vi "connect to arduino.vi"() -> ()   [LabVIEW 2020]
uses:
  <vilib>/Instr/_visa.llb/VISA Configure Serial Port (Instr).vi
panel:
  in  "mesurement period (ms)":dbl(slide) scale=0.0..2000.0
  out "console":string
  in  "Connection":bool
  out "Connection LED":bool
  in  "baud rate (9600)":u32=9600
  out "Waveform Chart":dbl(graph)
  in  "Voltage mesure":bool
  in  "Single voltage":bool
  in  "LED blink":bool
  in  "LED on/off":bool
  out "Voltage":dbl
  in  "VISA 1":refnum<visa-resource-name>
  in  "exit":bool
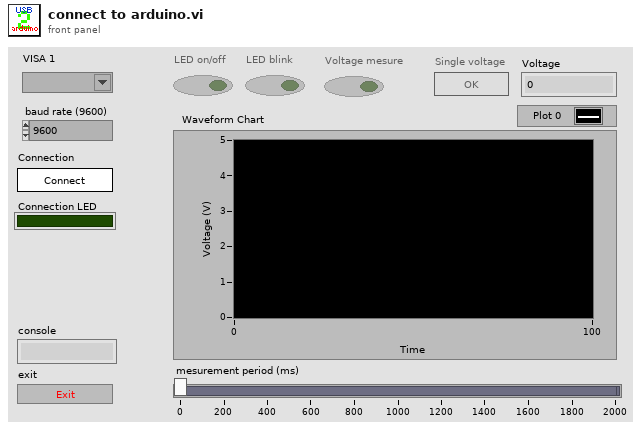
[diagram p1: front panel]
types:
  T1 = enum8{"Enabled", "Disabled", "Disabled and Grayed Out"}
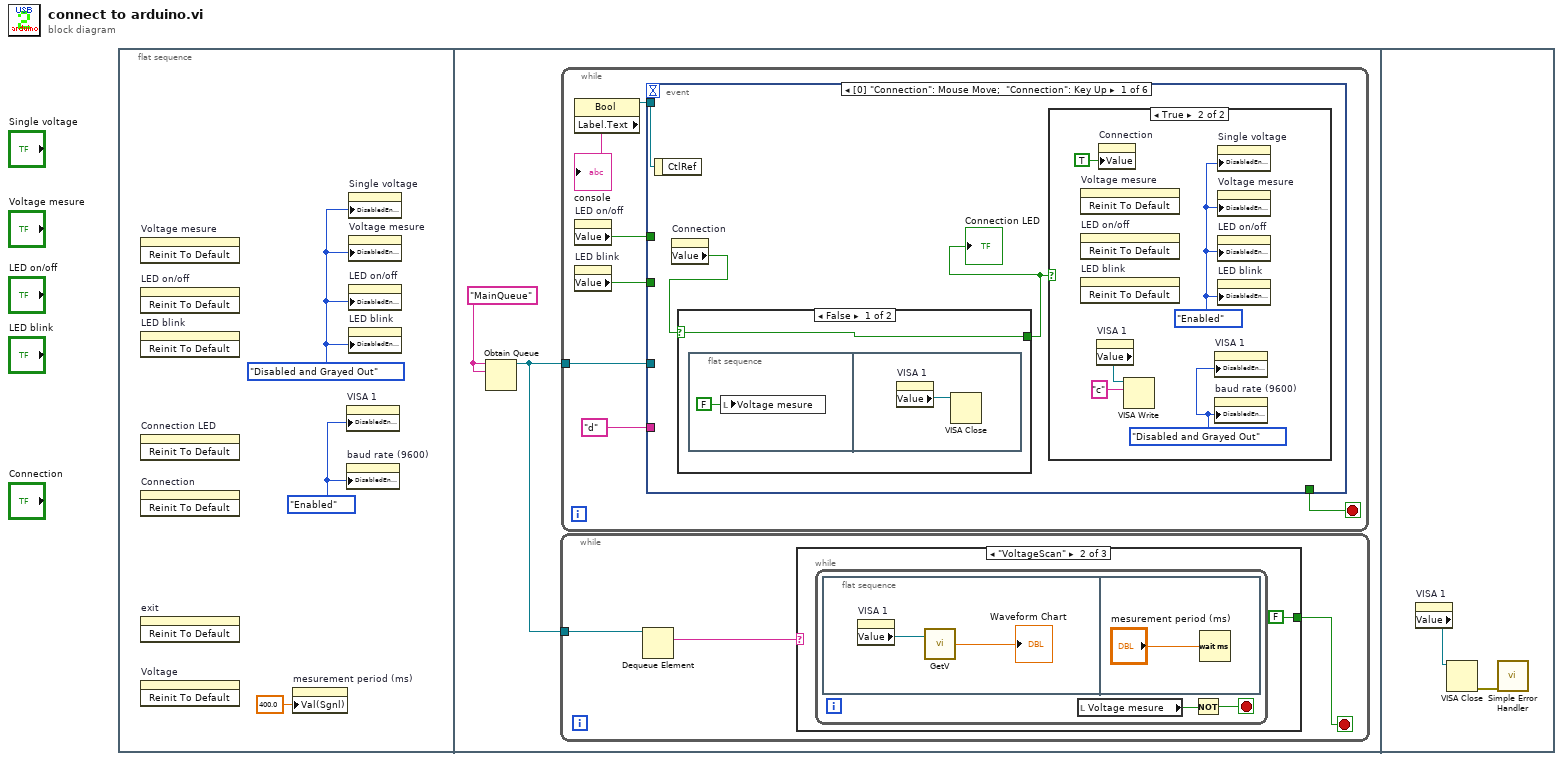
[diagram p0: block diagram]
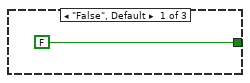
[diagram p2: hidden frame]
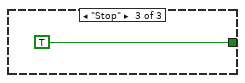
[diagram p3: hidden frame]
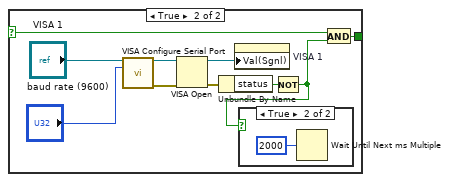
[diagram p4: hidden frame]
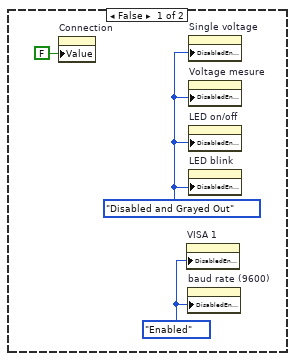
[diagram p6: hidden frame]
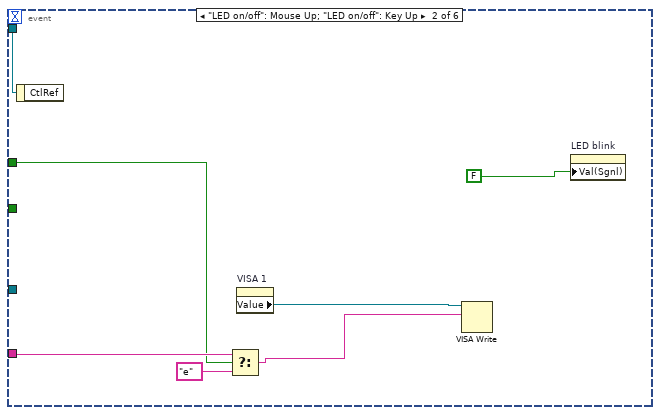
[diagram p7: hidden frame]
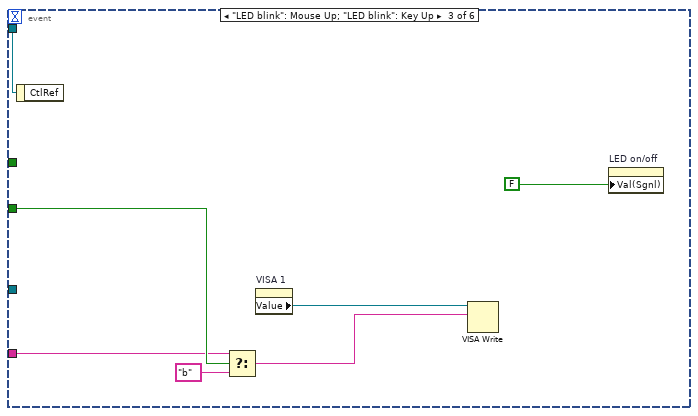
[diagram p8: hidden frame]
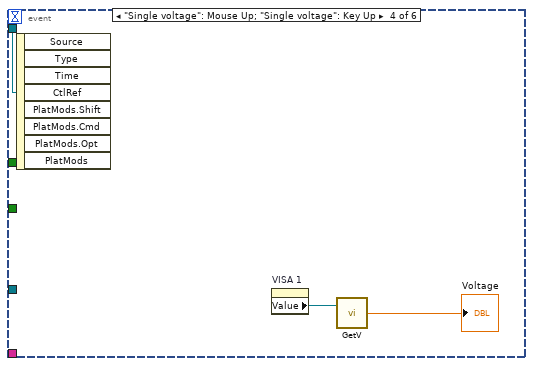
[diagram p9: hidden frame]
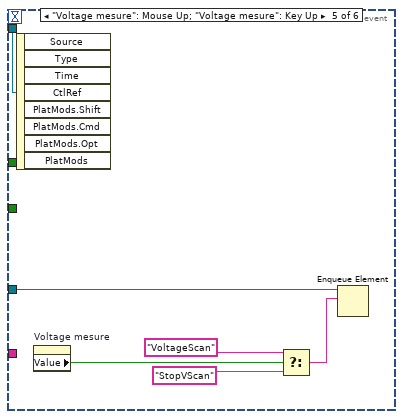
[diagram p10: hidden frame]
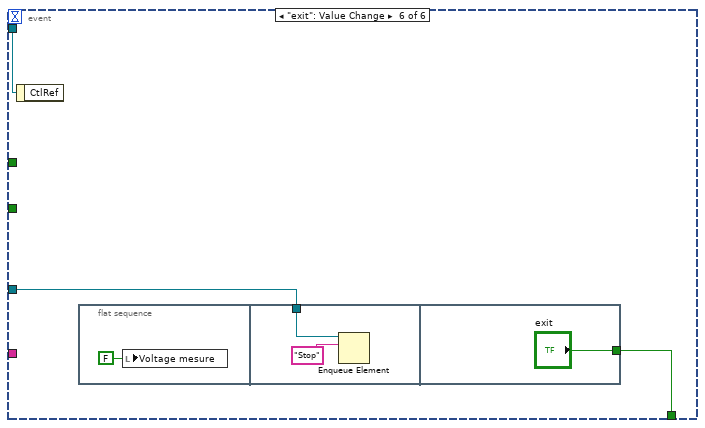
[diagram p11: hidden frame]
diagram:
  n1 = flat-sequence {
    frame #0 {
      w3 = T1."Enabled" ("Disabled")
      w2 = T1."Disabled and Grayed Out" ("Disabled")
      n2 = invoke on="Voltage mesure" class="Bool (strict)" method="Reinit To Default"() -> ()  [unwired: 3 in, 3 out]
      n3 = invoke on="LED on/off" class="Bool (strict)" method="Reinit To Default"() -> ()  [unwired: 3 in, 3 out]
      n4 = invoke on="LED blink" class="Bool (strict)" method="Reinit To Default"() -> ()  [unwired: 3 in, 3 out]
      n5 = invoke on="Connection LED" class="Bool (strict)" method="Reinit To Default"() -> ()  [unwired: 3 in, 3 out]
      n6 = invoke on="Connection" class="Bool (strict)" method="Reinit To Default"() -> ()  [unwired: 3 in, 3 out]
      n7 = invoke on="exit" class="Bool" method="Reinit To Default"() -> ()  [unwired: 3 in, 3 out]
      n8 = invoke on="Voltage" class="DigNum (strict)" method="Reinit To Default"() -> ()  [unwired: 3 in, 3 out]
      n9 = property on="mesurement period (ms)" class="Slide (strict)"("Val(Sgnl)"=400.0 ("Value (Signaling)")) -> ()  [unwired: 2 in, 2 out]
      n10 = property on="VISA 1" class="VISAName"("DisabledEnum"=w3) -> ()  [unwired: 2 in, 2 out]
      n11 = property on="baud rate (9600)" class="DigNum (strict)"("DisabledEnum"=w3) -> ()  [unwired: 2 in, 2 out]
      n12 = property on="Single voltage" class="Bool (strict)"("DisabledEnum"=w2) -> ()  [unwired: 2 in, 2 out]
      n13 = property on="Voltage mesure" class="Bool (strict)"("DisabledEnum"=w2) -> ()  [unwired: 2 in, 2 out]
      n14 = property on="LED on/off" class="Bool (strict)"("DisabledEnum"=w2) -> ()  [unwired: 2 in, 2 out]
      n15 = property on="LED blink" class="Bool (strict)"("DisabledEnum"=w2) -> ()  [unwired: 2 in, 2 out]
    }
    frame #1 {
      w5 = "MainQueue" ("name (unnamed)")
      n16 = Obtain Queue(name (unnamed)=w5, element data type=w5) -> (queue out=w4:refnum<queue>)  [unwired: 3 in, 2 out]
      n17 = while {
        tunnel: w4 -> [w6]
        stop <- w7 stop-if-true
        n18 = Dequeue Element(queue=w6) -> (element=w8:string)  [unwired: 2 in, 3 out]
        n19 = case shown="\"VoltageScan\"" w8 {
          tunnel: [FALSE FALSE TRUE] -> w7
          frame "False", Default {
          }
          frame "VoltageScan" {
            n20 = while {
              stop <- w12 stop-if-true
              n21 = flat-sequence {
                frame #0 {
                  n22 = property on="VISA 1" class="VISAName"() -> ("Value"=w13:refnum<visa-resource-name>)  [unwired: 2 in, 2 out]
                  n23 = call "GetV.vi"("VISA resource name"=w13) -> ("output 1"=→"Waveform Chart":dbl)  [unwired: 2 in, 1 out]
                }
                frame #1 {
                  n24 = Wait (ms)(milliseconds to wait="mesurement period (ms)") -> ()  [unwired: 1 out]
                }
              }
              n25 = local read "Voltage mesure"() -> (w11:bool)
              n26 = Not(x=w11) -> (.not. x?=w12:bool)
            }
          }
          frame "Stop" {
          }
        }
      }
      n27 = while {
        tunnel: w4 -> [w18]
        stop <- w17 stop-if-true
        n28 = property on="LED on/off" class="Bool (strict)"() -> ("Value"=w22:bool)  [unwired: 2 in, 2 out]
        n29 = property on="LED blink" class="Bool (strict)"() -> ("Value"=w21:bool)  [unwired: 2 in, 2 out]
        n30 = event shown="[0] \"Connection\": Mouse Move;  \"Connection\": Key Up" {
          selector: _ -> [_ _ _ _ _ _]
          dyn-events: _ -> [_ _ _ _ _ _]
          timeout: _ -> [_ _ _ _ _ _]
          tunnel: w22 -> [_ w52 _ _ _ _]
          tunnel: w21 -> [_ _ w61 _ _ _]
          tunnel: "d" -> [_ w54 w60 _ _ _]
          tunnel: [w26 w50 w57 w64 w70 w74] -> w19
          tunnel: [_ _ _ _ _ w73] -> w17
          tunnel: w18 -> [_ _ _ _ w71 w72]
          event "Connection": Mouse Move; "Connection": Key Up {
            n31 = event-data() -> ("CtlRef"=w26:refnum<vi>)  [unwired: 1 in]
            n32 = property on="Connection" class="Bool (strict)"() -> ("Value"=w25:bool)  [unwired: 2 in, 2 out]
            n33 = case shown="False" w25 {
              selector: w25 -> [w27 w33]
              tunnel: [w27 w34] -> w24
              frame False {
                n34 = flat-sequence {
                  frame #0 {
                    n35 = local write "Voltage mesure"(FALSE ("Voltage mesure")) -> ()
                  }
                  frame #1 {
                    n36 = property on="VISA 1" class="VISAName"() -> ("Value"=w29:refnum<visa-resource-name>)  [unwired: 2 in, 2 out]
                    n37 = VISA Close(VISA resource name=w29) -> ()  [unwired: 1 in, 1 out]
                  }
                }
              }
              frame True {
                n38 = call-poly "VISA Configure Serial Port"("VISA resource name"="VISA 1", "baud rate (9600)"="baud rate (9600)") -> ("VISA resource name out"=w36:refnum<visa-resource-name>, "error out"=w37:errorcluster)  [unwired: 12 in]
                n39 = VISA Open(error in (no error)=w37, VISA resource name=w36) -> (VISA resource name=w35:refnum<visa-resource-name>, error out=w31:errorcluster)  [unwired: 3 in]
                n40 = Unbundle By Name(w31) -> ("status"=w32:bool)
                n41 = property on="VISA 1" class="VISAName"("Val(Sgnl)"=w35) -> ()  [unwired: 2 in, 2 out]
                n42 = Not(x=w32) -> (.not. x?=w30:bool)
                n43 = case shown="True" w30 {
                  frame False {
                  }
                  frame True {
                    n44 = Wait Until Next ms Multiple(millisecond multiple=u32 2000) -> ()  [unwired: 1 out]
                  }
                }
                n45 = And(x=w33, y=w30) -> (x .and. y?=w34:bool)
              }
            }
            "Connection LED" <- w24
            n46 = case shown="True" w24 {
              frame False {
                w43 = T1."Enabled" ("Disabled")
                w42 = T1."Disabled and Grayed Out" ("Disabled")
                n47 = property on="Connection" class="Bool (strict)"("Value"=FALSE ("Connection")) -> ()  [unwired: 2 in, 2 out]
                n48 = property on="VISA 1" class="VISAName"("DisabledEnum"=w43) -> ()  [unwired: 2 in, 2 out]
                n49 = property on="baud rate (9600)" class="DigNum (strict)"("DisabledEnum"=w43) -> ()  [unwired: 2 in, 2 out]
                n50 = property on="Single voltage" class="Bool (strict)"("DisabledEnum"=w42) -> ()  [unwired: 2 in, 2 out]
                n51 = property on="Voltage mesure" class="Bool (strict)"("DisabledEnum"=w42) -> ()  [unwired: 2 in, 2 out]
                n52 = property on="LED on/off" class="Bool (strict)"("DisabledEnum"=w42) -> ()  [unwired: 2 in, 2 out]
                n53 = property on="LED blink" class="Bool (strict)"("DisabledEnum"=w42) -> ()  [unwired: 2 in, 2 out]
              }
              frame True {
                w47 = T1."Disabled and Grayed Out" ("Disabled")
                w48 = T1."Enabled" ("Disabled")
                n54 = invoke on="Voltage mesure" class="Bool (strict)" method="Reinit To Default"() -> ()  [unwired: 3 in, 3 out]
                n55 = invoke on="LED on/off" class="Bool (strict)" method="Reinit To Default"() -> ()  [unwired: 3 in, 3 out]
                n56 = invoke on="LED blink" class="Bool (strict)" method="Reinit To Default"() -> ()  [unwired: 3 in, 3 out]
                n57 = property on="VISA 1" class="VISAName"() -> ("Value"=w45:refnum<visa-resource-name>)  [unwired: 2 in, 2 out]
                n58 = property on="Connection" class="Bool (strict)"("Value"=TRUE ("Connection")) -> ()  [unwired: 2 in, 2 out]
                n59 = VISA Write(VISA resource name=w45, write buffer="c") -> ()  [unwired: 1 in, 3 out]
                n60 = property on="VISA 1" class="VISAName"("DisabledEnum"=w47) -> ()  [unwired: 2 in, 2 out]
                n61 = property on="baud rate (9600)" class="DigNum (strict)"("DisabledEnum"=w47) -> ()  [unwired: 2 in, 2 out]
                n62 = property on="Single voltage" class="Bool (strict)"("DisabledEnum"=w48) -> ()  [unwired: 2 in, 2 out]
                n63 = property on="Voltage mesure" class="Bool (strict)"("DisabledEnum"=w48) -> ()  [unwired: 2 in, 2 out]
                n64 = property on="LED on/off" class="Bool (strict)"("DisabledEnum"=w48) -> ()  [unwired: 2 in, 2 out]
                n65 = property on="LED blink" class="Bool (strict)"("DisabledEnum"=w48) -> ()  [unwired: 2 in, 2 out]
              }
            }
          }
          event "LED on/off": Mouse Up; "LED on/off": Key Up {
            n66 = event-data() -> ("CtlRef"=w50:refnum<vi>)  [unwired: 1 in]
            n67 = Select(t=w54, s=w52, f="e") -> (s? t:f=w51:string)
            n68 = property on="VISA 1" class="VISAName"() -> ("Value"=w49:refnum<visa-resource-name>)  [unwired: 2 in, 2 out]
            n69 = VISA Write(VISA resource name=w49, write buffer=w51) -> ()  [unwired: 1 in, 3 out]
            n70 = property on="LED blink" class="Bool (strict)"("Val(Sgnl)"=FALSE ("Value (Signaling)")) -> ()  [unwired: 2 in, 2 out]
          }
          event "LED blink": Mouse Up; "LED blink": Key Up {
            n71 = event-data() -> ("CtlRef"=w57:refnum<vi>)  [unwired: 1 in]
            n72 = Select(t=w60, s=w61, f="b") -> (s? t:f=w58:string)
            n73 = property on="VISA 1" class="VISAName"() -> ("Value"=w56:refnum<visa-resource-name>)  [unwired: 2 in, 2 out]
            n74 = VISA Write(VISA resource name=w56, write buffer=w58) -> ()  [unwired: 1 in, 3 out]
            n75 = property on="LED on/off" class="Bool (strict)"("Val(Sgnl)"=FALSE ("Value (Signaling)")) -> ()  [unwired: 2 in, 2 out]
          }
          event "Single voltage": Mouse Up; "Single voltage": Key Up {
            n76 = event-data() -> ("CtlRef"=w64:refnum<vi>)  [unwired: 1 in, 7 out]
            n77 = property on="VISA 1" class="VISAName"() -> ("Value"=w63:refnum<visa-resource-name>)  [unwired: 2 in, 2 out]
            n78 = call "GetV.vi"("VISA resource name"=w63) -> ("output 1"=→"Voltage":dbl)  [unwired: 2 in, 1 out]
          }
          event "Voltage mesure": Mouse Up; "Voltage mesure": Key Up {
            n79 = event-data() -> ("CtlRef"=w70:refnum<vi>)  [unwired: 1 in, 7 out]
            n80 = property on="Voltage mesure" class="Bool (strict)"() -> ("Value"=w68:bool)  [unwired: 2 in, 2 out]
            n81 = Select(t="VoltageScan" ("element"), s=w68, f="StopVScan" ("element")) -> (s? t:f=w69:string)
            n82 = Enqueue Element(queue=w71, element=w69) -> ()  [unwired: 2 in, 3 out]
          }
          event "exit": Value Change {
            n83 = event-data() -> ("CtlRef"=w74:refnum<vi>)  [unwired: 1 in]
            n84 = flat-sequence {
              tunnel: w72 -> [w76]
              tunnel: ["exit"] -> w73
              frame #0 {
                n85 = local write "Voltage mesure"(FALSE ("Voltage mesure")) -> ()
              }
              frame #1 {
                n86 = Enqueue Element(queue=w76, element="Stop") -> ()  [unwired: 2 in, 3 out]
              }
              frame #2 {
              }
            }
          }
        }
        n87 = property class="Bool"(reference=w19) -> ("Label.Text"=→"console":string)  [unwired: 1 in, 2 out]
      }
    }
    frame #2 {
      n88 = property on="VISA 1" class="VISAName"() -> ("Value"=w80:refnum<visa-resource-name>)  [unwired: 2 in, 2 out]
      n89 = VISA Close(VISA resource name=w80) -> (error out=w79:errorcluster)  [unwired: 1 in]
      n90 = call <vilib>:"Simple Error Handler.vi"("error in (no error)"=w79) -> ()  [unwired: 4 in, 5 out]
    }
  }
